vi "Exp01_GetOneData.vi"() -> ()   [LabVIEW 2019]
uses:
  <vilib>/myRIO/Instrument Drivers/Onboard IO/I2C/typedefs/I2C User Configuration.ctl
  <vilib>/myRIO/Instrument Drivers/Onboard IO/I2C/typedefs/I2C Transfer Rate.ctl
  <vilib>/Platform/TimedLoop/XDataNode/timing_clust.ctl
  <vilib>/Platform/TimedLoop/XDataNode/nitl_modes.ctl
  <vilib>/Platform/TimedLoop/XDataNode/wakeup.ctl
  <vilib>/Utility/error.llb/Error Cluster From Error Code.vi
  <vilib>/myRIO/Common/Instrument Driver Framework/myRIO v1.0/I2C/vis/myRIO v1.0 Configure I2C.vi
  <vilib>/myRIO/Common/Instrument Driver Framework/myRIO v1.0/I2C/vis/myRIO v1.0 Write I2C.vi
  <vilib>/myRIO/Common/Instrument Driver Framework/myRIO v1.0/I2C/vis/myRIO v1.0 Read I2C.vi
  <vilib>/Platform/TimedLoop/XDataNode/XDataNode.xnode
  <vilib>/myRIO/Instrument Drivers/Onboard IO/I2C/I2C.lvlib
  <vilib>/Platform/TimedLoop/XDataNode/XDNodeRunTimeDep.lvlib
panel:
  out "Bytes Read (decimal)":u8[](array[numeric]) format="%0d"
  out "Gyro Z":i16
  out "Gyro X":i16
  out "Gyro Y":i16
  out "Acc Z":i16
  out "Temperature":dbl
  out "Acc Y":i16
  out "Acc X":i16
  in  "stop":bool
  out "error out":errorcluster
  out "Bytes Read (binary)":u8[](array[numeric]) format="%08b"
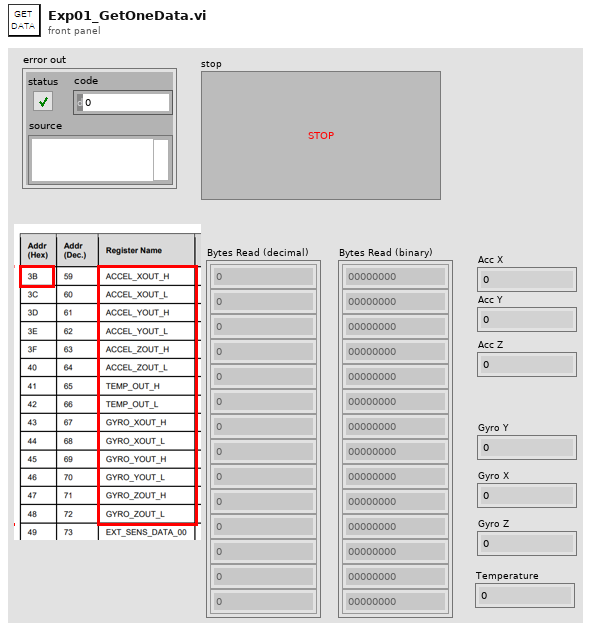
[diagram p1: front panel]
types:
  T1 = typedef "I2C.lvlib/I2C User Configuration.ctl" = cluster{"I2C Transfer Rate":T2}
  T2 = typedef "I2C.lvlib/I2C Transfer Rate.ctl" = enum16{"Standard mode (100 kbps)", "Fast mode (400 kbps)"}
  T3 = typedef "I2C.lvlib/I2C Reference.ctl" = cluster{"myRIO Reference":T4, "I2C Channels Enum":T8, "I2C Configuration":T9}
  T4 = typedef "myRIO Generic Hardware Reference.ctl" = cluster{"myRIO Model":T5, "myRIO Hardware Reference":T6}
  T5 = typedef "Hardware Version Enum.ctl" = enum16{"Unknown", "myRIO-1900", "myRIO-1950", "roboRIO", "NI ELVIS RIO CM", "ELVIS III"}
  T6 = typedef "myRIO v1.0 Reference.ctl" = cluster{"Generic FPGA Reference":T7, "Allow multiple opens":bool}
  T7 = typedef "Generic FPGA Reference.ctl" = refnum<k20>
  T8 = typedef "I2C Channels Enum.ctl" = enum16{"Not Connected", "A/I2C", "B/I2C", "I2C/I2C"}
  T9 = typedef "I2C.lvlib/I2C Configuration.ctl" = cluster{"I2C Transfer Rate":T2}
  T10 = typedef "XDNodeRunTimeDep.lvlib/timing_clust.ctl" = cluster{"Expected End [f-1]":u64, "Actual End [f-1]":u64, "Finished Late? [f-1]":bool, "Expected End [i-1]":u64, "Actual End [i-1]":u64, "Finished Late? [i-1]":bool, "Expected Start [i]":u64, "Actual Start [i]":u64, "Expected Start [f]":u64, "Actual Start [f]":u64, "Source Name":string, "Structure Name":string, "Period":i64, "Deadline":i64, "Offset":i64, "Start":i64, "Priority":i32, "Timeout":i32, "Mode":T11, "Wakeup Reason":T12, "Error":errorcluster, "Source Type":string, "Secondary Source Type":string, "Global End Time":u64, "Global Start Time":u64, "Frame Duration":u64, "Iteration Duration":u64, "Assigned CPU":i32, "I/O Scan Engine Mode":u32}
  T11 = typedef "XDNodeRunTimeDep.lvlib/nitl_modes.ctl" = enum32{"No Change", "Process missed periods, maintain original phase", "Discard missed periods, maintain original phase", "Process missed periods, ignore original phase", "Discard missed periods, ignore original phase"}
  T12 = typedef "XDNodeRunTimeDep.lvlib/wakeup.ctl" = enum32{"Normal", "Aborted", "Asynchronous wakeup", "Timing source error", "Timed loop error", "Timeout"}
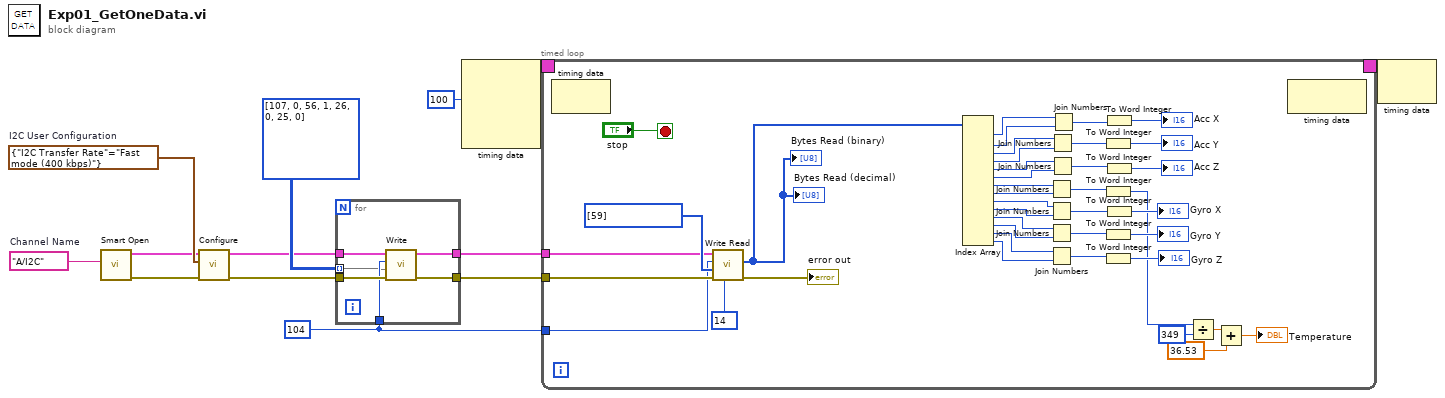
[diagram p0: block diagram]
diagram:
  w7 = u8 104 ("Slave Address (7-bit)")
  w12 = T1 {"I2C Transfer Rate"=enum."Fast mode (400 kbps)"}  # I2C User Configuration
  w13 = tag "A/I2C"  # Channel Name
  n1 = call <vilib>:"Smart Open.vi"("Channel Name"=w13) -> ("error out"=w10:errorcluster, "I2C Ref Out"=w11:T3)  [unwired: 9 in]
  n2 = call <vilib>:"Configure.vi"("error in (no error)"=w10, "I2C User Configuration"=w12, "I2C Ref In"=w11) -> ("error out"=w1:errorcluster, "I2C Ref Out"=w2:T3)  [unwired: 7 in]
  n3 = for {
    tunnel: w7 -> [w15]
    tunnel: w2 -> [w19]
    tunnel: [w16] -> w8
    tunnel: w1 -> [w18]
    tunnel: [w17] -> w9
    tunnel: u8[][] [[107, 0], [56, 1], [26, 0], [25, 0]] ("Bytes to Write") -> [w14] mode=indexing
    n4 = call <vilib>:"Write.vi"("error in (no error)"=w18, "Bytes to Write"=w14, "Slave Address (7-bit)"=w15, "I2C Ref In"=w19) -> ("error out"=w17:errorcluster, "I2C Ref Out"=w16:T3)  [unwired: 6 in]
  }
  n5 = node-c288(i64 100 ("Period")) -> (w6:T10)  [unwired: 3 in]
  n6 = timed-loop {
    timing: w6 -> [_]
    timing-out: [_] -> w5
    tunnel: w9 -> [w56]
    tunnel: w8 -> [w55]
    tunnel: w7 -> [w54]
    stop <- "stop" stop-if-true
    n7 = node-c288() -> ()  [unwired: 1 in, 1 out]
    n8 = call <vilib>:"Write Read.vi"("Byte Count"=u32 14, "error in (no error)"=w56, "Bytes to Write"=u8[] [59], "Slave Address (7-bit)"=w54, "I2C Ref In"=w55) -> ("error out"=→"error out":errorcluster, "Bytes Read"=w20:u8[])  [unwired: 3 in, 1 out]
    "Bytes Read (binary)" <- w20
    "Bytes Read (decimal)" <- w20
    n9 = Index Array(array=w20) -> (element #1=w52:u8, element #2=w51:u8, element #3=w50:u8, element #4=w49:u8, element #5=w48:u8, element #6=w47:u8, element #7=w46:u8, element #8=w45:u8, element #9=w44:u8, element #10=w43:u8, element #11=w42:u8, element #12=w41:u8, element #13=w40:u8, element #14=w39:u8)  [unwired: 14 in]
    n10 = Join Numbers(hi=w46, lo=w45) -> ((hi.lo)=w35:u16)
    n11 = Join Numbers(hi=w44, lo=w43) -> ((hi.lo)=w34:u16)
    n12 = Join Numbers(hi=w42, lo=w41) -> ((hi.lo)=w33:u16)
    n13 = Join Numbers(hi=w40, lo=w39) -> ((hi.lo)=w32:u16)
    n14 = Join Numbers(hi=w50, lo=w49) -> ((hi.lo)=w37:u16)
    n15 = Join Numbers(hi=w48, lo=w47) -> ((hi.lo)=w36:u16)
    n16 = Join Numbers(hi=w52, lo=w51) -> ((hi.lo)=w38:u16)
    n17 = To Word Integer(number=w37) -> (16bit integer=→"Acc Y":i16)
    n18 = To Word Integer(number=w35) -> (16bit integer=w25:i16)
    n19 = To Word Integer(number=w33) -> (16bit integer=→"Gyro Y":i16)
    n20 = To Word Integer(number=w32) -> (16bit integer=→"Gyro Z":i16)
    n21 = To Word Integer(number=w38) -> (16bit integer=→"Acc X":i16)
    n22 = To Word Integer(number=w36) -> (16bit integer=→"Acc Z":i16)
    n23 = To Word Integer(number=w34) -> (16bit integer=→"Gyro X":i16)
    n24 = Divide(x=w25, y=i16 349) -> (x/y=w23:dbl)
    n25 = Add(x=w23, y=36.53) -> (x+y=→"Temperature":dbl)
    n26 = node-c288() -> ()  [unwired: 1 in, 1 out]
  }
  n27 = node-c288(w5) -> ()  [unwired: 1 out]
